vi "Data Directory.vi"(11 "Subfolder (None)":path=path "") -> (3 "GCentral Data":path)   [LabVIEW 2020, in "GCentral-API.lvlib"]
uses:
  GCentral-API.lvlib
  <vilib>/Utility/sysdir.llb/System Directory Type.ctl
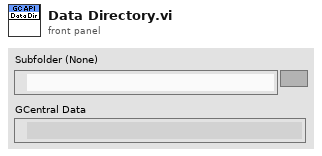
[diagram p1: front panel]
types:
  T1 = typedef "System Directory Type.ctl" = i32
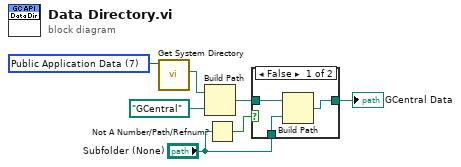
[diagram p0: block diagram]
diagram:
  w7 = T1 7 items=["User Home"=0, "User Desktop"=1, "User Documents"=2, "User Application Data"=3, "User Preferences"=4, "User Temporary"=5, "Public Documents"=6, "Public Application Data"=7, "Public Preferences"=8, "Public Cache"=13, "System Core Libraries"=9, "System Installed Libraries"=10, "Application Files"=11, "Boot Volume Root"=12] ("system directory type")
  n1 = call <vilib>:"Get System Directory.vi"("system directory type"=w7) -> ("system directory"=w6:path)  [unwired: 10 in]
  n2 = Build Path(base path=w6, name or relative path=path "GCentral") -> (appended path=w4:path)
  n3 = Not A Number/Path/Refnum?(number/path/refnum="Subfolder (None)") -> (NaN/Path/Refnum?=w3:bool)
  n4 = case shown="False" w3 {
    tunnel: w4 -> [w10 w11]
    tunnel: "Subfolder (None)" -> [w9 _]
    tunnel: [w8 w11] -> w1
    frame False {
      n5 = Build Path(base path=w10, name or relative path=w9) -> (appended path=w8:path)
    }
    frame True {
    }
  }
  "GCentral Data" <- w1
